vi "SetupEUIEvents.vi"(8 "error in (no error)":errorcluster, 11 "Model in":refnum<class "Model.lvclass">) -> (0 "error out":errorcluster, 3 "Model out":refnum<class "Model.lvclass">)   [LabVIEW 2016, in "Model.lvclass"]
uses:
  Model.lvclass
  EUI Events/EUI Events.lvclass
  Model.lvclass/Model.ctl
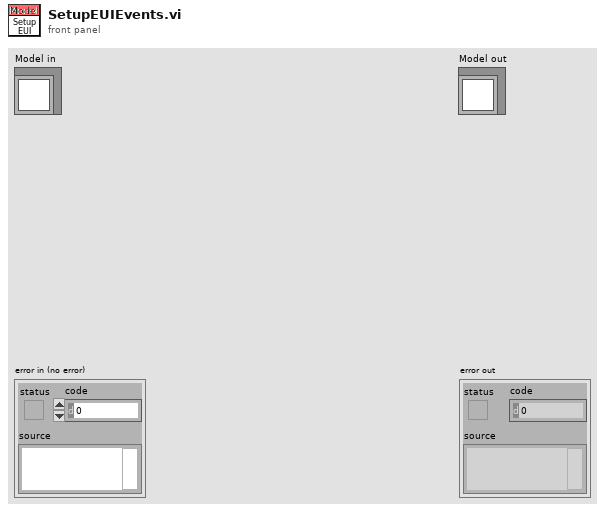
[diagram p1: front panel]
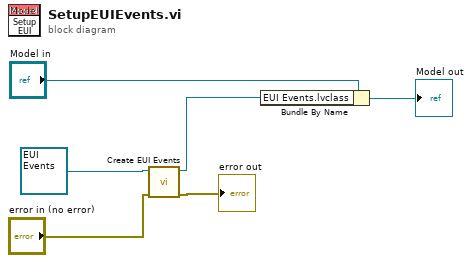
[diagram p0: block diagram]
diagram:
  n1 = call "Create EUI Events.vi"("error in (no error)"="error in (no error)", "EUI Events in"=refnum<class "EUI Events.lvclass"> refnum ("EUI Events.lvclass")) -> ("error out"=→"error out":errorcluster, "EUI Events out"=w2:refnum<class "EUI Events.lvclass">)  [unwired: 8 in]
  n2 = Bundle By Name(cluster="Model in", "EUI Events.lvclass"=w2) -> (→"Model out":refnum<class "Model.lvclass">)
